vi "Pack For Grpc.vi"(8 "error in (no error)":errorcluster, 9 "Configuration / Resuls (Config)":enum16{"Configuration", "Results"}(ring), 10 "Data Value":variant, 11 "Measurement Customizations in":refnum<class "MeasurementPlugin.lvclass">) -> (0 "error out":errorcluster, 2 "Any":T1, 3 "Measurement Customizations out":refnum<class "MeasurementPlugin.lvclass">)   [LabVIEW 2020, in "NIDCPowerSourceDCVoltage.lvlib" / "MeasurementPlugin.lvclass"]
uses:
  MeasurementPlugin.lvclass
  <vilib>/gRPC/LabVIEW gRPC Library/Shared/Any.ctl
  Measurement Configuration.ctl
  Measurement Results.ctl
  2eca732d-dbaa-43bf-a7dd-ede2da65bc1b.vi
  a6012965-5700-4384-8228-972e71b6560c.vi
  <vilib>/gRPC/LabVIEW gRPC Library/Server API/Translate Protobuf Error.vi
  <vilib>/AdvancedString/1D String Array to Delimited String.vi
  <vilib>/gRPC/LabVIEW gRPC Library/Server API/Server/Get Server DLL Path.vi
  NIDCPowerSourceDCVoltage.lvlib
  <vilib>/gRPC/LabVIEW gRPC Library/grpc-lvsupport-release.lvlib
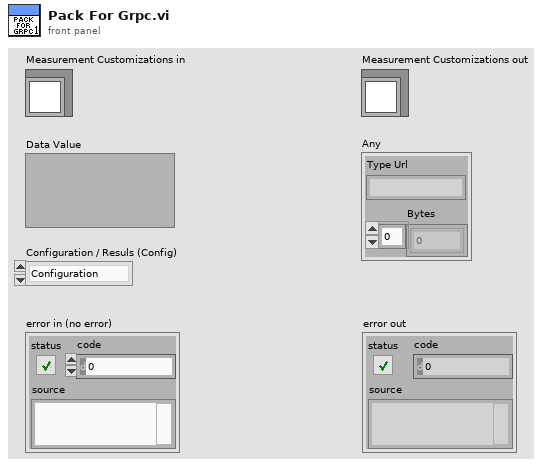
[diagram p1: front panel]
types:
  T1 = typedef "grpc-lvsupport-release.lvlib/Any.ctl" = cluster{"Type Url":string, "Bytes":u8[]}
  T2 = typedef "grpc-lvsupport-release.lvlib/grpcId.ctl" = u64
  T3 = typedef "NIDCPowerSourceDCVoltage.lvlib/Measurement Configuration.ctl" = cluster{"pin_names":string[], "voltage_level":dbl, "voltage_level_range":dbl, "current_limit":dbl, "current_limit_range":dbl, "source_delay":dbl}
  T4 = typedef "NIDCPowerSourceDCVoltage.lvlib/Measurement Results.ctl" = cluster{"measurement_sites":i32[], "measurement_pin_names":string[], "voltage_measurements":dbl[], "current_measurements":dbl[], "in_compliance":bool[]}
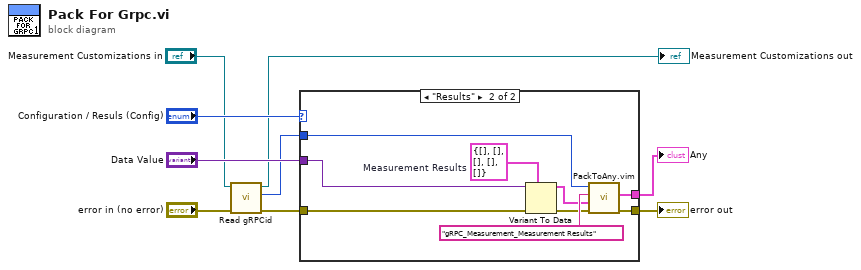
[diagram p0: block diagram]
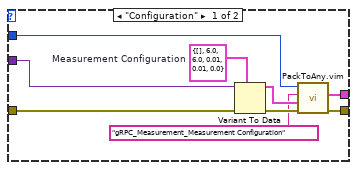
[diagram p2: hidden frame]
diagram:
  n1 = call-dynamic "Read gRPCid.vi"("error in"="error in (no error)", "iService in"="Measurement Customizations in") -> ("error out"=w4:errorcluster, "gRPCid"=w1:T2, "iService out"=→"Measurement Customizations out":refnum<class "MeasurementPlugin.lvclass">)  [unwired: 7 in]
  n2 = case shown="\"Results\"" "Configuration / Resuls (Config)" {
    tunnel: w4 -> [w18 w27]
    tunnel: "Data Value" -> [w17 w26]
    tunnel: w1 -> [w14 w22]
    tunnel: [w16 w24] -> w8
    tunnel: [w15 w23] -> w7
    frame "Configuration" {
      w11 = T3 {"pin_names"=[], "voltage_level"=6.0, "voltage_level_range"=6.0, "current_limit"=0.01, "current_limit_range"=0.01, "source_delay"=0.0}  # Measurement Configuration
      n3 = Variant To Data(error in=w18, type=w11, Variant=w17) -> (data=w13:T3, error out=w12:errorcluster)
      n4 = call "PackToAny.vim"("error in"=w12, "Data To Pack"=w13, "Message Type"="gRPC_Measurement_Measurement Configuration", "gRPCid in"=w14) -> ("error out"=w16:errorcluster, "Any"=w15:T1)  [unwired: 5 in, 1 out]
    }
    frame "Results" {
      w25 = T4 {"measurement_sites"=[], "measurement_pin_names"=[], "voltage_measurements"=[], "current_measurements"=[], "in_compliance"=[]}  # Measurement Results
      n5 = Variant To Data(error in=w27, type=w25, Variant=w26) -> (data=w20:T4, error out=w19:errorcluster)
      n6 = call "PackToAny.vim"("error in"=w19, "Data To Pack"=w20, "Message Type"="gRPC_Measurement_Measurement Results", "gRPCid in"=w22) -> ("error out"=w24:errorcluster, "Any"=w23:T1)  [unwired: 5 in, 1 out]
    }
  }
  "error out" <- w8
  "Any" <- w7
